vi "ATF-Device channel list.vi"(7 "Enum":enum16{"Read", "Write"}(ring), 8 "error in (no error)":errorcluster, 10 "Device List":T2, 11 "Channel List":T1) -> (0 "error out":errorcluster, 2 "Device List R":T2, 3 "Channel List R":T1)   [LabVIEW 2022 SP3]
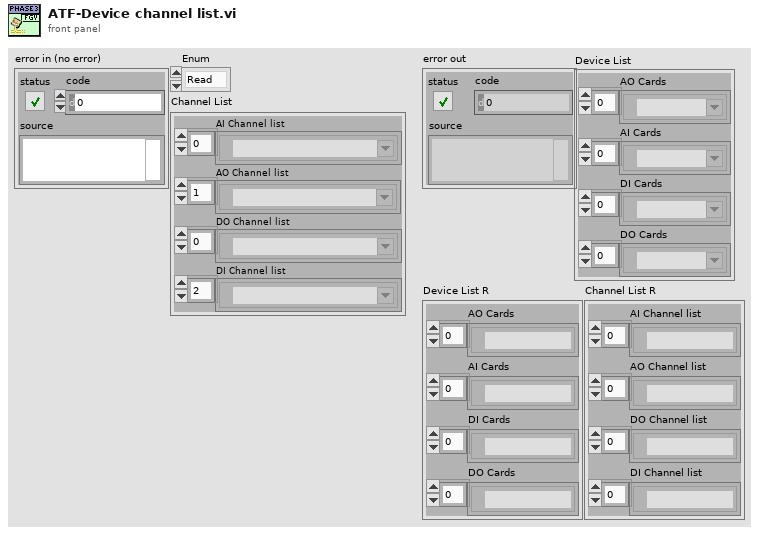
[diagram p1: front panel]
types:
  T1 = cluster{"AI Channel list":tag[], "AO Channel list":tag[], "DO Channel list ":tag[], "DI Channel list":tag[]}
  T2 = cluster{"AO Cards":tag[], "AI Cards":tag[], "DI Cards":tag[], "DO Cards":tag[]}
  T3 = cluster{"Device List":cluster{"AO Cards":tag[], "AI Cards":tag[], "DI Cards":tag[], "DO Cards":tag[]}, "Channel List":cluster{"AI Channel list":tag[], "AO Channel list":tag[], "DO Channel list ":tag[], "DI Channel list":tag[]}}
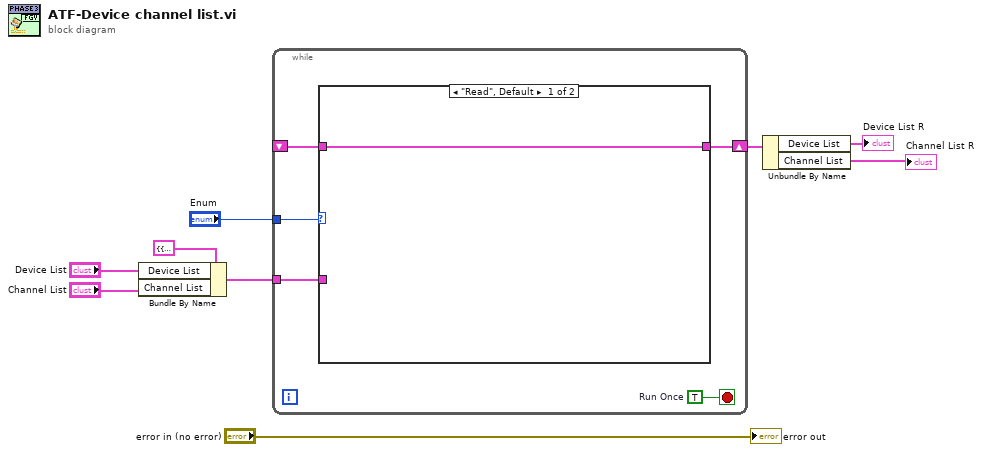
[diagram p0: block diagram]
diagram:
  n1 = Bundle By Name(cluster=T3 {"Device List"={"AO Cards"=[], "AI Cards"=[], "DI Cards"=[], "DO Cards"=[]}, "Channel List"={"AI Channel list"=[], "AO Channel list"=[], "DO Channel list "=[], "DI Channel list"=[]}}, "Device List"="Device List", "Channel List"="Channel List") -> (w4:T3)
  n2 = while {
    shift-right: [w10] -> w3
    shift-left: _ -> [w13]
    tunnel: "Enum" -> [w12]
    tunnel: w4 -> [w11]
    stop <- w14 stop-if-true
    w14 = TRUE  # Run Once
    n3 = case shown="\"Read\", Default" w12 {
      tunnel: w13 -> [w15 _]
      tunnel: w11 -> [_ w16]
      tunnel: [w15 w16] -> w10
      frame "Read", Default {
      }
      frame "Write" {
      }
    }
  }
  n4 = Unbundle By Name(w3) -> ("Device List"=→"Device List R":T2, "Channel List"=→"Channel List R":T1)
  "error out" <- "error in (no error)"
